vi "logger_data.vi"(10 "data_store_mode":enum16{"Set", "Get"}(ring), 11 "dashboard_data":T12={"gun_fast"={"speed_setpoint"=0.0, "speed_sensor"=0.0, "gun_power"=0.0, "gun_control_mode"=enum."Hold Power", "gun_tracking_mode"=enum."manual_aim"}, "gun_slow"={"turret"={"turret_analog"=0.0, "turret_angle"=0.0, "turret_motor"=0.0, "turret_idg_state"=enum."fault_high"}, "hood"={"hood_analog"=0.0, "hood_angle"=0.0, "hood_motor"=0.0, "hood_idg_state"=enum."fault_high"}}, "drivetrain_data"={"left"={"request"=0.0, "enc_speed"=0.0}, "right"={"request"=0.0, "enc_speed"=0.0}, "gear shift state"=enum."low", "gear shift internal state"=enum."low"}, "roller data"={"roller internal state"=enum."idle", "roller user state"=enum."off", "sws"={"r_sw_b1"=FALSE, "r_sw_b2"=FALSE, "r_sw_b3"=FALSE, "r_sw_gun"=FALSE, "r_sw_low"=FALSE}}, "joe_johnson_data"={"analog"=0.0, "input"=0.0, "joe_johnson_state"=enum."fold", "idg_state"=enum."fault_high"}}) -> (3 "dashboard_data_out":T12={"gun_fast"={"speed_setpoint"=0.0, "speed_sensor"=0.0, "gun_power"=0.0, "gun_control_mode"=enum."Hold Power", "gun_tracking_mode"=enum."manual_aim"}, "gun_slow"={"turret"={"turret_analog"=0.0, "turret_angle"=0.0, "turret_motor"=0.0, "turret_idg_state"=enum."fault_high"}, "hood"={"hood_analog"=0.0, "hood_angle"=0.0, "hood_motor"=0.0, "hood_idg_state"=enum."fault_high"}}, "drivetrain_data"={"left"={"request"=0.0, "enc_speed"=0.0}, "right"={"request"=0.0, "enc_speed"=0.0}, "gear shift state"=enum."low", "gear shift internal state"=enum."low"}, "roller data"={"roller internal state"=enum."idle", "roller user state"=enum."off", "sws"={"r_sw_b1"=FALSE, "r_sw_b2"=FALSE, "r_sw_b3"=FALSE, "r_sw_gun"=FALSE, "r_sw_low"=FALSE}}, "joe_johnson_data"={"analog"=0.0, "input"=0.0, "joe_johnson_state"=enum."fold", "idg_state"=enum."fault_high"}})   [LabVIEW 2011]
uses:
  dashboard_data_gun_fast.ctl
  gun/gun_motor_state.ctl
  gun/gun_tracking_mode.ctl
  gun/gun_rt_slow_upstream_data.ctl
  idg_trust_t.ctl
  dashboard_data_drivetrain.ctl
  drivetrain/gear_shift_state.ctl
  drivetrain/gear_internal_shift_state.ctl
  roller/roller_internal_state.ctl
  roller/roller_user_state.ctl
  joe_johnson/joe_johnson_state.ctl
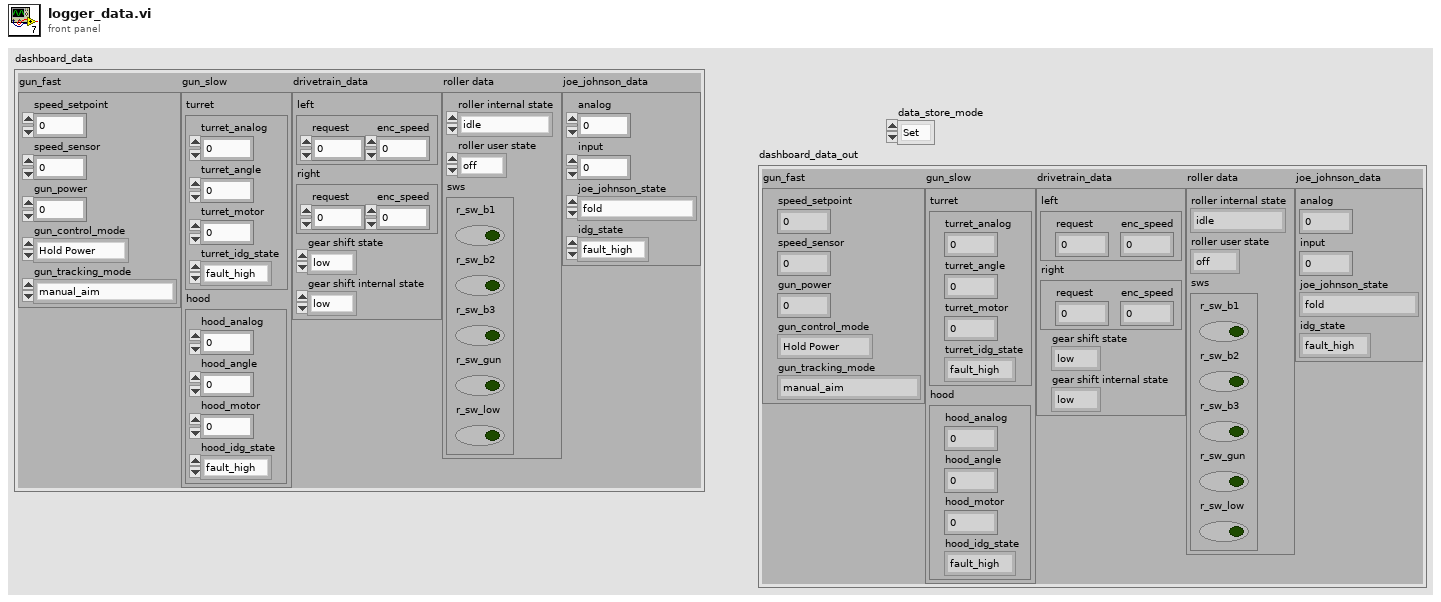
[diagram p1: front panel]
types:
  T1 = typedef "dashboard_data_gun_fast.ctl" = cluster{"speed_setpoint":dbl, "speed_sensor":dbl, "gun_power":dbl, "gun_control_mode":T2, "gun_tracking_mode":T3}
  T2 = typedef "gun_motor_state.ctl" = enum16{"Hold Power", "Hold Speed", "Hold Distance", "Stop"}
  T3 = typedef "gun_tracking_mode.ctl" = enum16{"manual_aim", "auto_aim_camera", "preset_center_field", "preset_right_pocket", "preset_left_pocket", "align_center", "align_center_backwards", "auto_aim_key", "align_fold", "auton_custom", "preset_pass", "auto_aim_auton"}
  T4 = typedef "gun_rt_slow_upstream_data.ctl" = cluster{"turret":cluster{"turret_analog":dbl, "turret_angle":dbl, "turret_motor":dbl, "turret_idg_state":T5}, "hood":cluster{"hood_analog":dbl, "hood_angle":dbl, "hood_motor":dbl, "hood_idg_state":T5}}
  T5 = typedef "idg_trust_t.ctl" = enum16{"fault_move", "fault_high", "fault_low", "out_high", "out_low", "trust"}
  T6 = typedef "dashboard_data_drivetrain.ctl" = cluster{"left":cluster{"request":dbl, "enc_speed":dbl}, "right":cluster{"request":dbl, "enc_speed":dbl}, "gear shift state":T7, "gear shift internal state":T8}
  T7 = typedef "gear_shift_state.ctl" = enum16{"low", "high"}
  T8 = typedef "gear_internal_shift_state.ctl" = enum16{"low", "high", "low_peak", "high_peak"}
  T9 = typedef "roller_internal_state.ctl" = enum16{"idle", "bump", "full", "fire_intermediate", "fire_finish", "fire_entry", "fire_end", "fire_recover"}
  T10 = typedef "roller_user_state.ctl" = enum16{"off", "collect", "blow", "force suck"}
  T11 = typedef "joe_johnson_state.ctl" = enum16{"fold", "down", "up", "ramp", "bridge_lift", "manual", "ramp_stay"}
  T12 = cluster{"gun_fast":T1, "gun_slow":T4, "drivetrain_data":T6, "roller data":cluster{"roller internal state":T9, "roller user state":T10, "sws":cluster{"r_sw_b1":bool, "r_sw_b2":bool, "r_sw_b3":bool, "r_sw_gun":bool, "r_sw_low":bool}}, "joe_johnson_data":cluster{"analog":dbl, "input":dbl, "joe_johnson_state":T11, "idg_state":T5}}
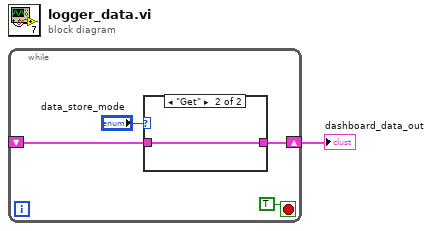
[diagram p0: block diagram]
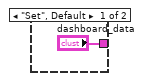
[diagram p2: hidden frame]
diagram:
  n1 = while {
    shift-right: [w3] -> w1
    shift-left: _ -> [w2]
    stop <- TRUE stop-if-true
    n2 = case shown="\"Get\"" "data_store_mode" {
      tunnel: ["dashboard_data" w7] -> w3
      tunnel: w2 -> [_ w7]
      frame "Set", Default {
      }
      frame "Get" {
      }
    }
  }
  "dashboard_data_out" <- w1
